vi "Run (non-indexed).vi"(8 "error in (no error)":errorcluster, 10 "States LUT (name -> boolean state)":variant, 11 "TriggerAction in":refnum<class "TriggerAction Q.lvclass">) -> (0 "error out":errorcluster, 3 "TriggerAction out":refnum<class "TriggerAction Q.lvclass">)   [LabVIEW 2016, in "TriggerAction Q.lvclass"]
uses:
  <userlib>/Common Components/TriggerAction Q/TriggerAction Q/TriggerAction Q.lvclass
  <userlib>/Common Components/TriggerAction Q/TriggerAction Q/TriggerAction Q.lvclass/TriggerAction Q.ctl
  <userlib>/Common Components/Function Messages/Action Dispatch Msg/Action Dispatch Msg.lvclass/Action Dispatch Msg.ctl
  <vilib>/ActorFramework/Message Enqueuer/Message Enqueuer.lvclass/Message Enqueuer.ctl
  <vilib>/ActorFramework/Message Enqueuer/Enqueue.vi
  <userlib>/Common Components/Function Messages/Action Dispatch Msg/Action Dispatch Msg.lvclass
  C:/Program Files (x86)/National Instruments/LabVIEW 2016/vi.lib/ActorFramework/Message/Message.lvclass
  <vilib>/ActorFramework/Message Priority Queue/Priority Enqueue.vi
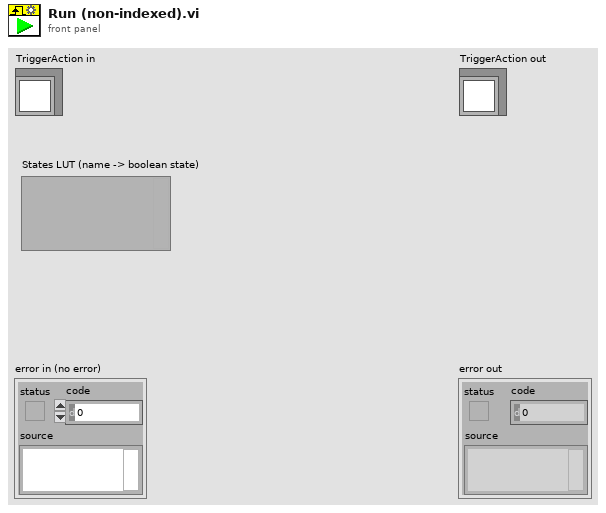
[diagram p1: front panel]
types:
  T1 = typedef "TriggerAction.lvclass/Element Data.ctl" = cluster{"Triggers":cluster{"Triggers for Array AND":string[]}[], "Actions":cluster{"Action Name":string, "Action Data":string}[]}
  T2 = cluster{"Action Name":string, "Action Data":string}[]
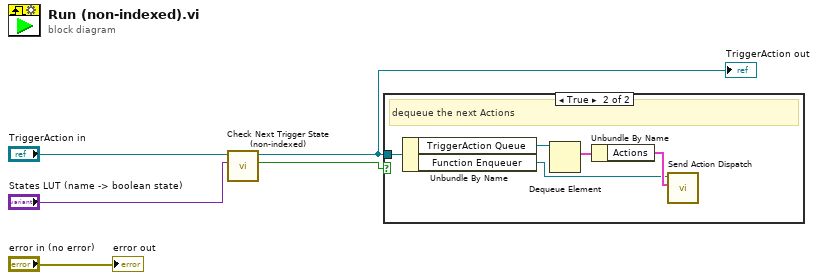
[diagram p0: block diagram]
diagram:
  n1 = call <userlib>:"Check Next Trigger State (non-indexed).vi"("States LUT (name -> boolean state)"="States LUT (name -> boolean state)", "TriggerAction in"="TriggerAction in") -> ("Trigger State"=w3:bool, "TriggerAction out"=w2:refnum<class "TriggerAction Q.lvclass">)  [unwired: 7 in, 1 out]
  "TriggerAction out" <- w2
  n2 = case shown="True" w3 {
    tunnel: w2 -> [_ w10]
    frame False {
    }
    frame True {
      # "dequeue the next Actions"
      n3 = Unbundle By Name(w10) -> ("TriggerAction Queue"=w9:refnum<queue>, "Function Enqueuer"=w6:refnum<class "Message Enqueuer.lvclass">)
      n4 = Dequeue Element(queue=w9) -> (element=w8:T1)  [unwired: 2 in, 3 out]
      n5 = Unbundle By Name(w8) -> ("Actions"=w7:T2)
      n6 = call <userlib>:"Send Action Dispatch.vi"("Actions"=w7, "Message Enqueuer"=w6) -> ()  [unwired: 8 in, 2 out]
    }
  }
  "error out" <- "error in (no error)"
